vi "Do.vi"(8 "error in (no error)":errorcluster, 10 "Actor in":refnum<class "Actor.lvclass">, 11 "Set F Start Parameter Msg":refnum<class "Set F Start Parameter Msg.lvclass">) -> (0 "error out":errorcluster, 2 "Actor out":refnum<class "Actor.lvclass">)   [LabVIEW 2014, in "HIJ Vision Fluence Cam.lvlib" / "Set F Start Parameter Msg.lvclass"]
doc: "This VI delivers the message to the actor by calling the appropriate method(s) on the actor."
uses:
  Set F Start Parameter Msg.lvclass
  <vilib>/ActorFramework/Actor/Actor.lvclass
  Launcher/HIJ Vision Fluence Cam Launcher.lvclass
  Set F Start Parameter Msg.lvclass/Set F Start Parameter Msg.ctl
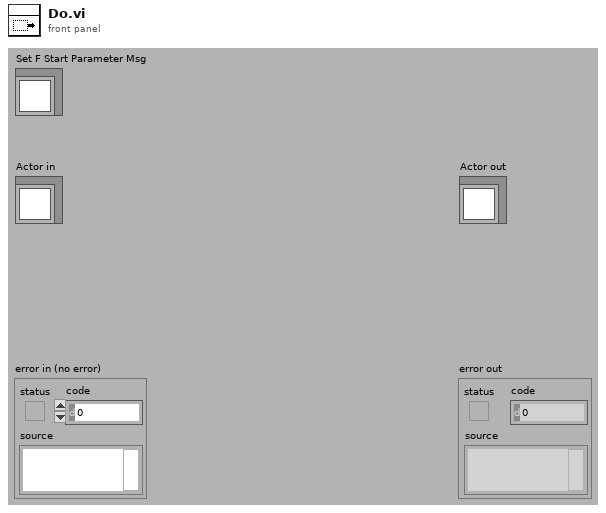
[diagram p1: front panel]
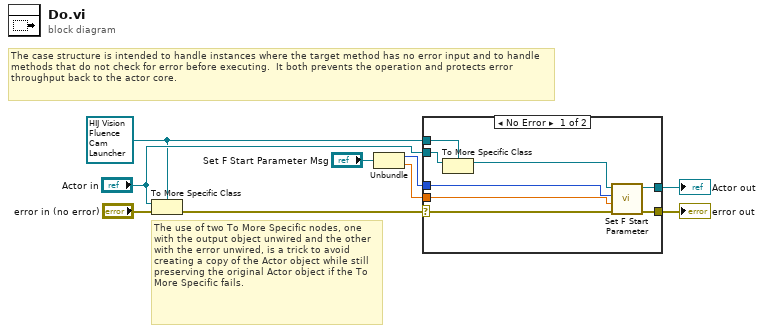
[diagram p0: block diagram]
diagram:
  w3 = refnum<class "HIJ Vision Fluence Cam Launcher.lvclass"> refnum ("Actor in")
  # "The use of two To More Specific nodes, one with the output object unwired and the other with the error unwired, is a trick to avoid creating a copy of the Actor object while still preserving the original Actor object if the To More Specific fails."
  # "The case structure is intended to handle instances where the target method has no error input and to handle methods that do not check for error before executing.  It both prevents the operation and protects error throughput back to the actor core."
  n1 = To More Specific Class(target class=w3, reference="Actor in", error in="error in (no error)") -> (error out=w7:errorcluster)  [unwired: 1 out]
  n2 = Unbundle("Set F Start Parameter Msg") -> (w2:u8, w1:dbl[unit])
  n3 = case shown="No Error" w7 {
    selector: w7 -> [w15 w19]
    tunnel: [w17 w19] -> w6
    tunnel: [w16 w18] -> w5
    tunnel: "Actor in" -> [w14 w18]
    tunnel: w3 -> [w13 _]
    tunnel: w2 -> [w11 _]
    tunnel: w1 -> [w10 _]
    frame No Error {
      n4 = To More Specific Class(target class=w13, reference=w14) -> (specific class reference=w12:refnum<class "HIJ Vision Fluence Cam Launcher.lvclass">)  [unwired: 1 in, 1 out]
      n5 = call "Set F Start Parameter.vi"("error in (no error)"=w15, "@Energy"=w10, "Size of Region"=w11, "HIJ Vision Fluence Cam Launcher in"=w12) -> ("error out"=w17:errorcluster, "HIJ Vision Fluence Cam Launcher out"=w16:refnum<class "HIJ Vision Fluence Cam Launcher.lvclass">)  [unwired: 6 in]
    }
    frame Error {
      # "If type check fails, pass the original object out again."
    }
  }
  "error out" <- w6
  "Actor out" <- w5
